vi "ConvertBooleanToSCPIValue.vi"(11 "Boolean":bool) -> (3 "SCPI Value":string)   [LabVIEW 8.6, in "Keithley-6482-Visa.lvlib"]
uses:
  Keithley-6482-Visa.lvlib
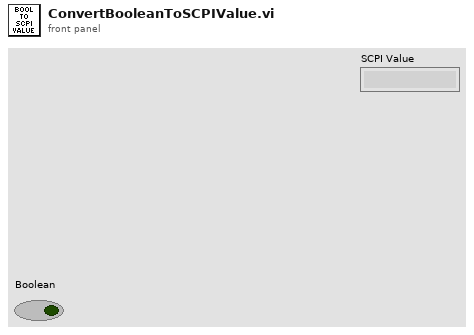
[diagram p1: front panel]
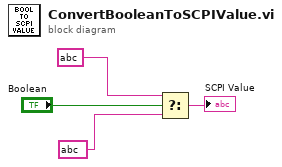
[diagram p0: block diagram]
diagram:
  n1 = Select(t=string ?, s="Boolean", f=string ?) -> (s? t:f=→"SCPI Value":string)
